vi "单个流程写入.vi"(7 "添加的路径":path, 8 "error in (no error)":errorcluster caption="错误输入（无错误）", 9 "量程":enum16{"低量程", "高量程"}(ring), 10 "测量模式":u16(ring) items=["", "水样测量", "标样核查", "零点核查", "跨度核查", "空白测试", "平行样测试", "加标回收", "填充管路", "清洗管路", "清洗反应杯"], 11 "测量参数":u16(ring)=21 items=["总磷"=0, "总氮"=1, "CODMn"=21]) -> (0 "error out":errorcluster caption="错误输出", 3 "步数":i32)   [LabVIEW 2016]
panel:
  out "数组 2":u16[][](array[numeric]) format="0x%04x"
  out "大小":i32
  out "交织的数组":u16[](array[numeric]) format="0x%04x"
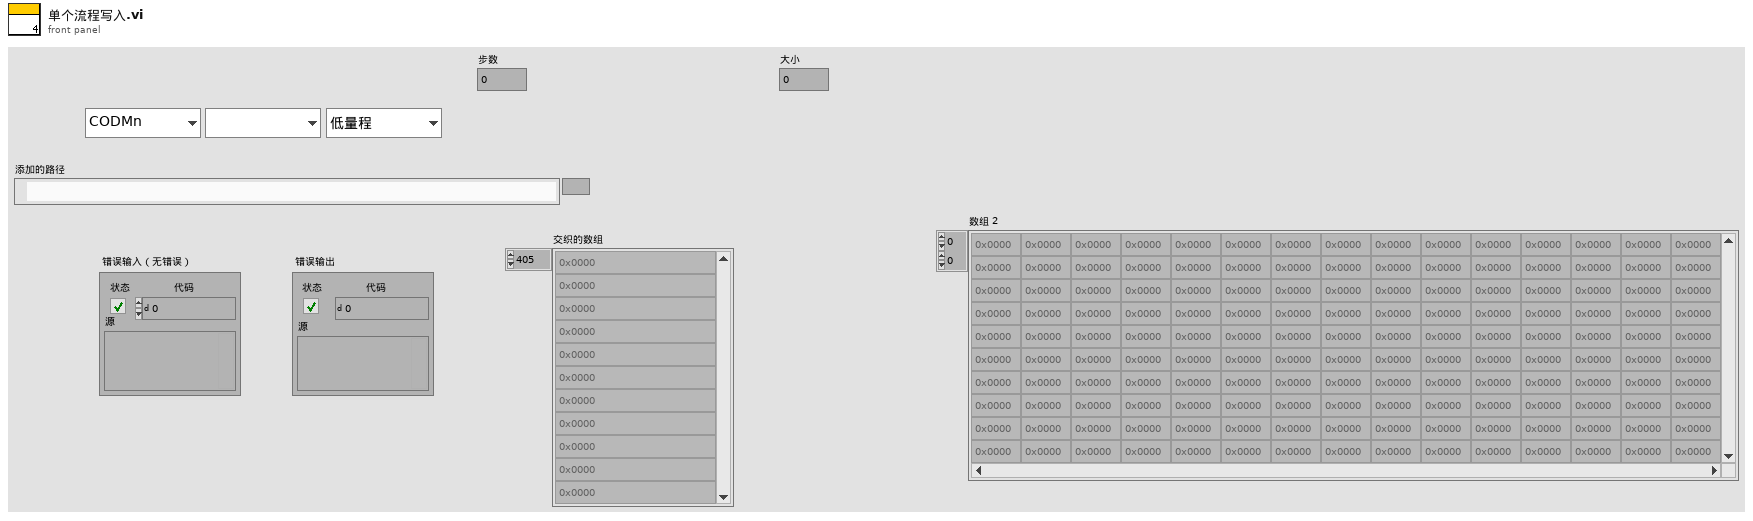
[diagram p1: front panel]
types:
  T1 = cluster{"站号":u16, "starting address":u16, "starting address":u16}
  T2 = cluster{"port":u32, "pump":u16, "temp":u8, "adc":u8, "time":u16, "步骤名":string}[]
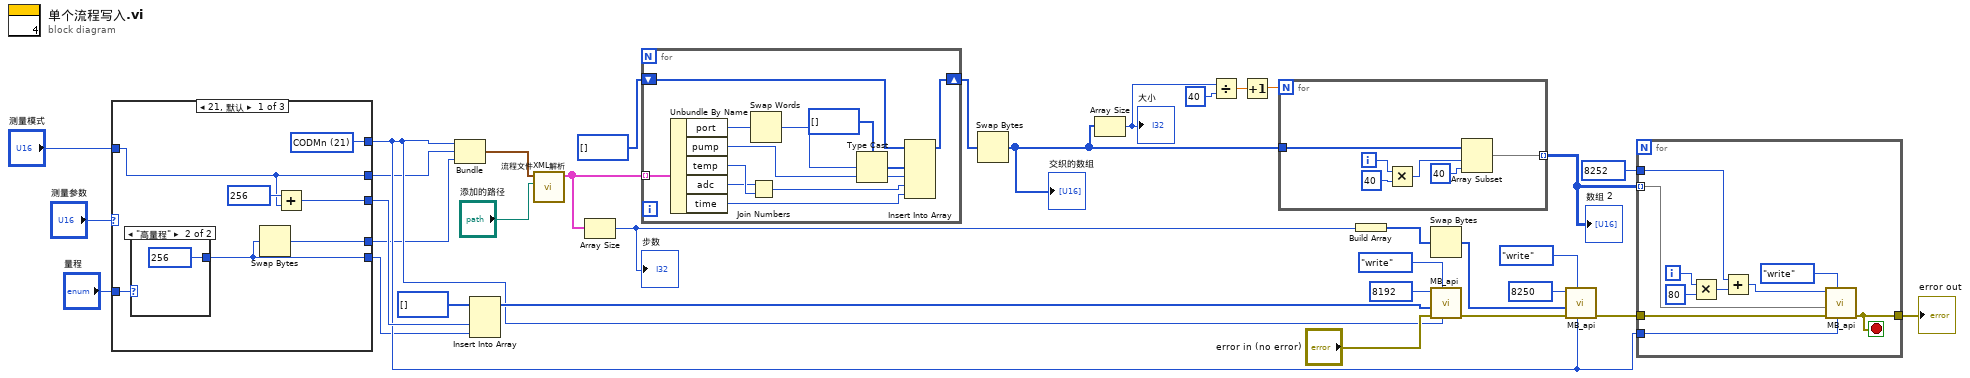
[diagram p0: block diagram]
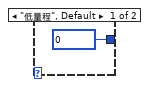
[diagram p2: hidden frame]
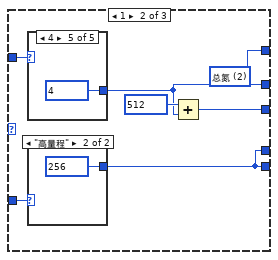
[diagram p3: hidden frame]
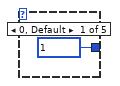
[diagram p4: hidden frame]
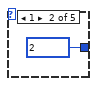
[diagram p5: hidden frame]
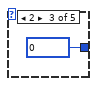
[diagram p6: hidden frame]
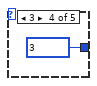
[diagram p7: hidden frame]
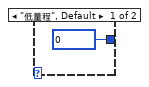
[diagram p8: hidden frame]
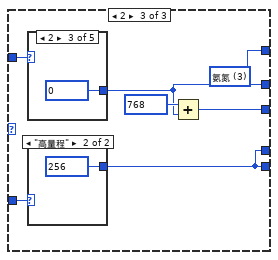
[diagram p9: hidden frame]
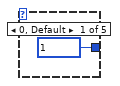
[diagram p10: hidden frame]
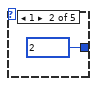
[diagram p11: hidden frame]
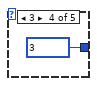
[diagram p12: hidden frame]
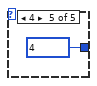
[diagram p13: hidden frame]
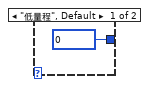
[diagram p14: hidden frame]
diagram:
  n1 = case shown="21, 默认" "测量参数" {
    tunnel: "测量模式" -> [w36 w47 w61]
    tunnel: "量程" -> [w40 w48 w62]
    tunnel: [w37 w49 w63] -> w4
    tunnel: [w38 w45 w59] -> w29
    tunnel: [w35 w43 w57] -> w2
    tunnel: [w36 w44 w58] -> w3
    tunnel: [w34 w43 w57] -> w1
    frame 21, Default {
      w37 = u16 21 items=["CODMn"=21, "总氮"=2, "氨氮"=3] ("站号")
      n2 = case shown="\"高量程\"" w40 {
        tunnel: [u16 0 ("starting address") u16 256 ("starting address")] -> w35
        frame "低量程", Default {
        }
        frame "高量程" {
        }
      }
      n3 = Swap Bytes(anything=w35) -> (byte swapped=w34:u16)
      n4 = Add(x=u16 256 ("starting address"), y=w36) -> (x+y=w38:u16)
    }
    frame 1 {
      w49 = u16 2 items=["总磷"=1, "总氮"=2, "氨氮"=3] ("站号")
      n5 = case shown="4" w47 {
        tunnel: [u16 1 ("starting address") u16 2 ("starting address") u16 0 ("starting address") u16 3 ("starting address") u16 4 ("starting address")] -> w44
        frame 0, Default {
        }
        frame 1 {
        }
        frame 2 {
        }
        frame 3 {
        }
        frame 4 {
        }
      }
      n6 = case shown="\"高量程\"" w48 {
        tunnel: [u16 0 ("starting address") u16 256 ("starting address")] -> w43
        frame "低量程", Default {
        }
        frame "高量程" {
        }
      }
      n7 = Add(x=u16 512 ("starting address"), y=w44) -> (x+y=w45:u16)
    }
    frame 2 {
      w63 = u16 3 items=["总磷"=1, "总氮"=2, "氨氮"=3] ("站号")
      n8 = case shown="2" w61 {
        tunnel: [u16 1 ("starting address") u16 2 ("starting address") u16 0 ("starting address") u16 3 ("starting address") u16 4 ("starting address")] -> w58
        frame 0, Default {
        }
        frame 1 {
        }
        frame 2 {
        }
        frame 3 {
        }
        frame 4 {
        }
      }
      n9 = case shown="\"高量程\"" w62 {
        tunnel: [u16 0 ("starting address") u16 256 ("starting address")] -> w57
        frame "低量程", Default {
        }
        frame "高量程" {
        }
      }
      n10 = Add(x=u16 768 ("starting address"), y=w58) -> (x+y=w59:u16)
    }
  }
  n11 = Bundle("站号"=w4, "starting address"=w3, "starting address"=w1) -> (w5:T1)  [unwired: 1 in]
  n12 = Insert Into Array(array=u16[] [] ("数组"), new element #1=w29, new element #2=w2) -> (w23:u16[])  [unwired: 1 in]
  n13 = call "流程文件XML解析.vi"("添加的路径"="添加的路径", "参数簇"=w5) -> ("数组"=w12:T2)  [unwired: 9 in]
  n14 = Array Size(array=w12) -> (size(s)=w7:i32)
  "步数" <- w7
  n15 = for {
    tunnel: w12 -> [w82] mode=indexing
    shift-right: [w80] -> w17
    shift-left: u16[] [] -> [w78]
    n16 = Unbundle By Name(w82) -> ("port"=w75:u32, "pump"=w73:u16, "temp"=w77:u8, "adc"=w76:u8, "time"=w71:u16)
    n17 = Join Numbers(hi=w76, lo=w77) -> ((hi.lo)=w72:u16)
    n18 = Swap Words(1:w75) -> (0:w74:u32)
    n19 = Type Cast(type=u16[] [], x=w74) -> (*(type *) &x=w79:u16[])
    n20 = Insert Into Array(array=w78, new element #1=w79, new element #2=w73, new element #3=w72, new element #4=w71) -> (w80:u16[])  [unwired: 1 in]
  }
  n21 = Swap Bytes(anything=w17) -> (byte swapped=w14:u16[])
  "交织的数组" <- w14
  n22 = Array Size(array=w14) -> (size(s)=w16:i32)
  "大小" <- w16
  n23 = Divide(x=w16, y=40) -> (x/y=w10:dbl)
  n24 = Increment(x=w10) -> (x+1=w9:dbl)
  n25 = for {
    N: w9 -> [_]
    tunnel: w14 -> [w86]
    tunnel: [w83] -> w13 mode=indexing
    i -> [w88]
    n26 = Multiply(x=w88, y=40) -> (x*y=w85:i32)
    n27 = Array Subset(array=w86, index=w85, length=40 ("y")) -> (w83:u16[])
  }
  "数组 2" <- w13
  n28 = Build Array(w7) -> (w11:i32[])
  n29 = Swap Bytes(anything=w11) -> (byte swapped=w8:i32[])
  n30 = call "MB_api.vi"("Slave ID"=w4, "STEP"=enum16{"open", "read", "write", "close"}."write", "Error in"="error in (no error)", "values"=w23, "starting address"=u16 8192) -> ("error out"=w26:errorcluster)  [unwired: 4 in, 2 out]
  n31 = call "MB_api.vi"("Slave ID"=w4, "STEP"=enum16{"open", "read", "write", "close"}."write", "Error in"=w26, "values"=w8, "starting address"=u16 8250) -> ("error out"=w22:errorcluster)  [unwired: 4 in, 2 out]
  n32 = for {
    tunnel: u16 8252 ("starting address") -> [w92]
    tunnel: w22 -> [w98]
    tunnel: [w96] -> w20
    tunnel: w4 -> [w95]
    tunnel: w13 -> [w94] mode=indexing
    i -> [w91]
    stop <- w96 stop-if-true
    n33 = Multiply(x=w91, y=80) -> (x*y=w90:i32)
    n34 = Add(x=w92, y=w90) -> (x+y=w93:i32)
    n35 = call "MB_api.vi"("Slave ID"=w95, "STEP"=enum16{"open", "read", "write", "close"}."write", "Error in"=w98, "values"=w94, "starting address"=w93) -> ("error out"=w96:errorcluster)  [unwired: 4 in, 2 out]
  }
  "error out" <- w20
